vi "PDLM_AllDllFunctions_UIThread.vi"   [LabVIEW 2010]
uses:
  pdlm_lib_x86_x64_UIThread.llb/PDLM_DllPath_global.vi
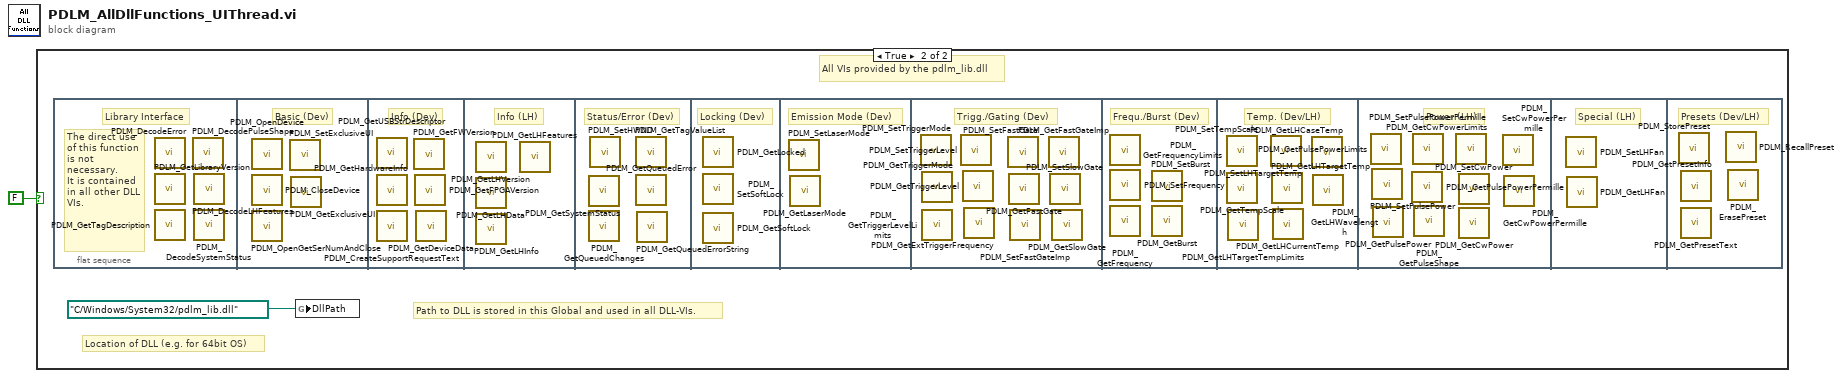
[diagram p0: block diagram]
diagram:
  n1 = case shown="True" FALSE {
    frame False {
    }
    frame True {
      # "Location of DLL (e.g. for 64bit OS)"
      # "Path to DLL is stored in this Global and used in all DLL-VIs."
      # "All VIs provided by the pdlm_lib.dll"
      n2 = flat-sequence {
        frame #0 {
          # "The direct use of this function is not necessary.\nIt is contained in all other DLL VIs."
          # "Library Interface"
          n3 = call "PDLM_DecodeError.vi"() -> ()  [unwired: 9 in, 3 out]
          n4 = call "PDLM_GetLibraryVersion.vi"() -> ()  [unwired: 9 in, 3 out]
          n5 = call "PDLM_GetTagDescription.vi"() -> ()  [unwired: 8 in, 4 out]
          n6 = call "PDLM_DecodePulseShape.vi"() -> ()  [unwired: 9 in, 3 out]
          n7 = call "PDLM_DecodeLHFeatures.vi"() -> ()  [unwired: 9 in, 3 out]
          n8 = call "PDLM_DecodeSystemStatus.vi"() -> ()  [unwired: 9 in, 3 out]
        }
        frame #1 {
          # "Basic (Dev)"
          n9 = call "PDLM_OpenDevice.vi"() -> ()  [unwired: 9 in, 3 out]
          n10 = call "PDLM_CloseDevice.vi"() -> ()  [unwired: 10 in, 2 out]
          n11 = call "PDLM_OpenGetSerNumAndClose.vi"() -> ()  [unwired: 9 in, 3 out]
          n12 = call "PDLM_SetExclusiveUI.vi"() -> ()  [unwired: 10 in, 2 out]
          n13 = call "PDLM_GetExclusiveUI.vi"() -> ()  [unwired: 9 in, 3 out]
        }
        frame #2 {
          # "Info (Dev)"
          n14 = call "PDLM_GetUSBStrDescriptor.vi"() -> ()  [unwired: 9 in, 3 out]
          n15 = call "PDLM_GetHardwareInfo.vi"() -> ()  [unwired: 9 in, 3 out]
          n16 = call "PDLM_CreateSupportRequestText.vi"() -> ()  [unwired: 9 in, 3 out]
          n17 = call "PDLM_GetFWVersion.vi"() -> ()  [unwired: 9 in, 3 out]
          n18 = call "PDLM_GetFPGAVersion.vi"() -> ()  [unwired: 9 in, 3 out]
          n19 = call "PDLM_GetDeviceData.vi"() -> ()  [unwired: 9 in, 3 out]
        }
        frame #3 {
          # "Info (LH)"
          n20 = call "PDLM_GetLHVersion.vi"() -> ()  [unwired: 9 in, 3 out]
          n21 = call "PDLM_GetLHData.vi"() -> ()  [unwired: 9 in, 3 out]
          n22 = call "PDLM_GetLHInfo.vi"() -> ()  [unwired: 9 in, 3 out]
          n23 = call "PDLM_GetLHFeatures.vi"() -> ()  [unwired: 9 in, 3 out]
        }
        frame #4 {
          # "Status/Error (Dev)"
          n24 = call "PDLM_GetSystemStatus.vi"() -> ()  [unwired: 9 in, 3 out]
          n25 = call "PDLM_GetQueuedChanges.vi"() -> ()  [unwired: 8 in, 4 out]
          n26 = call "PDLM_SetHWND.vi"() -> ()  [unwired: 10 in, 2 out]
          n27 = call "PDLM_GetTagValueList.vi"() -> ()  [unwired: 9 in, 3 out]
          n28 = call "PDLM_GetQueuedError.vi"() -> ()  [unwired: 9 in, 3 out]
          n29 = call "PDLM_GetQueuedErrorString.vi"() -> ()  [unwired: 9 in, 3 out]
        }
        frame #5 {
          # "Locking (Dev)"
          n30 = call "PDLM_GetLocked.vi"() -> ()  [unwired: 9 in, 3 out]
          n31 = call "PDLM_SetSoftLock.vi"() -> ()  [unwired: 10 in, 2 out]
          n32 = call "PDLM_GetSoftLock.vi"() -> ()  [unwired: 9 in, 3 out]
        }
        frame #6 {
          # "Emission Mode (Dev)"
          n33 = call "PDLM_SetLaserMode.vi"() -> ()  [unwired: 10 in, 2 out]
          n34 = call "PDLM_GetLaserMode.vi"() -> ()  [unwired: 9 in, 3 out]
        }
        frame #7 {
          # "Trigg./Gating (Dev)"
          n35 = call "PDLM_SetTriggerMode.vi"() -> ()  [unwired: 10 in, 2 out]
          n36 = call "PDLM_GetTriggerMode.vi"() -> ()  [unwired: 9 in, 3 out]
          n37 = call "PDLM_GetTriggerLevelLimits.vi"() -> ()  [unwired: 8 in, 4 out]
          n38 = call "PDLM_SetTriggerLevel.vi"() -> ()  [unwired: 10 in, 2 out]
          n39 = call "PDLM_GetTriggerLevel.vi"() -> ()  [unwired: 9 in, 3 out]
          n40 = call "PDLM_GetExtTriggerFrequency.vi"() -> ()  [unwired: 9 in, 3 out]
          n41 = call "PDLM_SetFastGate.vi"() -> ()  [unwired: 10 in, 2 out]
          n42 = call "PDLM_GetFastGate.vi"() -> ()  [unwired: 9 in, 3 out]
          n43 = call "PDLM_SetFastGateImp.vi"() -> ()  [unwired: 10 in, 2 out]
          n44 = call "PDLM_GetFastGateImp.vi"() -> ()  [unwired: 9 in, 3 out]
          n45 = call "PDLM_SetSlowGate.vi"() -> ()  [unwired: 10 in, 2 out]
          n46 = call "PDLM_GetSlowGate.vi"() -> ()  [unwired: 9 in, 3 out]
        }
        frame #8 {
          # "Frequ./Burst (Dev)"
          n47 = call "PDLM_GetFrequencyLimits.vi"() -> ()  [unwired: 8 in, 4 out]
          n48 = call "PDLM_SetFrequency.vi"() -> ()  [unwired: 10 in, 2 out]
          n49 = call "PDLM_GetFrequency.vi"() -> ()  [unwired: 9 in, 3 out]
          n50 = call "PDLM_SetBurst.vi"() -> ()  [unwired: 10 in, 2 out]
          n51 = call "PDLM_GetBurst.vi"() -> ()  [unwired: 8 in, 4 out]
        }
        frame #9 {
          # "Temp. (Dev/LH)"
          n52 = call "PDLM_SetTempScale.vi"() -> ()  [unwired: 10 in, 2 out]
          n53 = call "PDLM_GetTempScale.vi"() -> ()  [unwired: 9 in, 3 out]
          n54 = call "PDLM_GetLHTargetTempLimits.vi"() -> ()  [unwired: 8 in, 4 out]
          n55 = call "PDLM_SetLHTargetTemp.vi"() -> ()  [unwired: 10 in, 2 out]
          n56 = call "PDLM_GetLHTargetTemp.vi"() -> ()  [unwired: 9 in, 3 out]
          n57 = call "PDLM_GetLHCurrentTemp.vi"() -> ()  [unwired: 9 in, 3 out]
          n58 = call "PDLM_GetLHCaseTemp.vi"() -> ()  [unwired: 9 in, 3 out]
          n59 = call "PDLM_GetLHWavelength.vi"() -> ()  [unwired: 9 in, 3 out]
        }
        frame #10 {
          # "Power (LH)"
          n60 = call "PDLM_GetPulsePowerLimits.vi"() -> ()  [unwired: 8 in, 4 out]
          n61 = call "PDLM_SetPulsePower.vi"() -> ()  [unwired: 10 in, 2 out]
          n62 = call "PDLM_GetPulsePower.vi"() -> ()  [unwired: 9 in, 3 out]
          n63 = call "PDLM_GetPulsePowerPermille.vi"() -> ()  [unwired: 9 in, 3 out]
          n64 = call "PDLM_SetPulsePowerPermille.vi"() -> ()  [unwired: 10 in, 2 out]
          n65 = call "PDLM_GetPulseShape.vi"() -> ()  [unwired: 9 in, 3 out]
          n66 = call "PDLM_GetCwPowerLimits.vi"() -> ()  [unwired: 8 in, 4 out]
          n67 = call "PDLM_SetCwPower.vi"() -> ()  [unwired: 10 in, 2 out]
          n68 = call "PDLM_GetCwPower.vi"() -> ()  [unwired: 9 in, 3 out]
          n69 = call "PDLM_SetCwPowerPermille.vi"() -> ()  [unwired: 10 in, 2 out]
          n70 = call "PDLM_GetCwPowerPermille.vi"() -> ()  [unwired: 9 in, 3 out]
        }
        frame #11 {
          # "Special (LH)"
          n71 = call "PDLM_SetLHFan.vi"() -> ()  [unwired: 10 in, 2 out]
          n72 = call "PDLM_GetLHFan.vi"() -> ()  [unwired: 9 in, 3 out]
        }
        frame #12 {
          # "Presets (Dev/LH)"
          n73 = call "PDLM_StorePreset.vi"() -> ()  [unwired: 10 in, 2 out]
          n74 = call "PDLM_GetPresetInfo.vi"() -> ()  [unwired: 9 in, 3 out]
          n75 = call "PDLM_GetPresetText.vi"() -> ()  [unwired: 9 in, 3 out]
          n76 = call "PDLM_RecallPreset.vi"() -> ()  [unwired: 10 in, 2 out]
          n77 = call "PDLM_ErasePreset.vi"() -> ()  [unwired: 10 in, 2 out]
        }
      }
      n78 = global write "PDLM_DllPath_global.vi" "DllPath"(path "C:/Windows/System32/pdlm_lib.dll" ("DllPath")) -> ()
    }
  }
